vi "Test Get Documentation String.vi"() -> ()   [LabVIEW 2020]
uses:
  source/JKI SM/JKI SM.lvclass
panel:
  out "Documentation":string
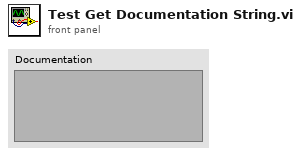
[diagram p1: front panel]
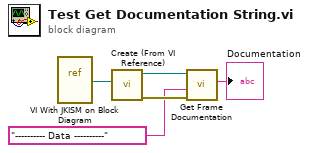
[diagram p0: block diagram]
diagram:
  n1 = vi-ref "VI With JKISM on Block Diagram.vi"() -> (w5:refnum<vi>)
  n2 = call "Create (From VI Reference).vi"("VI"=w5) -> ("error out"=w3:errorcluster, "JKI SM out"=w4:refnum<class "JKI SM.lvclass">)  [unwired: 9 in]
  n3 = call "Get Frame Documentation.vi"("error in (no error)"=w3, "State Name"="---------- Data ----------", "JKI SM in"=w4) -> ("Documentation"=→"Documentation":string)  [unwired: 6 in, 2 out]
